vi "Save-Load Non-profile values.vi"(6 "Which file? (User profile.ini)":T1=enum."Loaded User profile.ini", 8 "error in":errorcluster, 11 "Function":T2=enum."Load from file") -> (0 "error out":errorcluster)   [LabVIEW 2017]
uses:
  Typedefs/Save-Load enum.ctl
  Typedefs/Which path.ctl
  <vilib>/Utility/config.llb/NI_LVConfig.lvlib
panel:
  out "any found?":bool
  out "all found?":bool
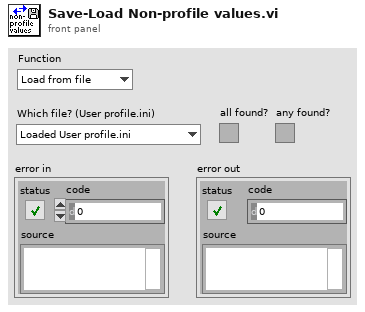
[diagram p1: front panel]
types:
  T1 = typedef "Which path.ctl" = enum16{"Configuration Files", "Calibration Files", "Images", "Setup.ini", "Loaded User profile.ini", "User's-Previous session.ini", "New user profile.ini", "Selected User profile.ini", "User profiles folder", "Power meter scaling.txt", "FOV Cal.ini"}
  T2 = typedef "Save-Load enum.ctl" = enum16{"Save to file", "Load from file", "Compare from file"}
  T3 = typedef "NI_LVConfig.lvlib/Config Data RefNum.ctl" = refnum<k1>
  T4 = typedef "Non-profile parameters cluster.ctl" = cluster{"Laser wavelength (nm)-When profile was saved":dbl}
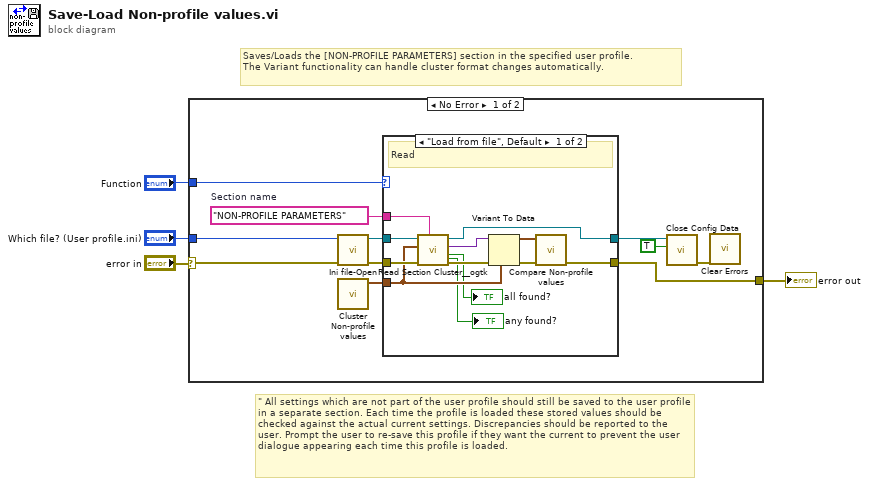
[diagram p0: block diagram]
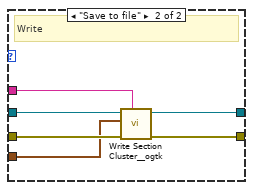
[diagram p2: hidden frame]
diagram:
  # "\"\tAll settings which are not part of the user profile should still be saved to the user profile in a separate section. Each time the profile is loaded these stored values should be checked against the actual current settings. Discrepancies should be reported to the user. Prompt the user to re-save this profile if they want the current to prevent the user dialogue appearing each time this profile is loaded."
  # "Saves/Loads the [NON-PROFILE PARAMETERS] section in the specified user profile.\nThe Variant functionality can handle cluster format changes automatically."
  n1 = case shown="No Error" "error in" {
    selector: "error in" -> [w6 w34]
    tunnel: [w8 w34] -> w4
    tunnel: "Which file? (User profile.ini)" -> [w9 _]
    tunnel: "Function" -> [w5 _]
    frame No Error {
      w15 = "NON-PROFILE PARAMETERS"  # Section name
      n2 = call "Ini file-Open.vi"("Error In"=w6, "Which file?"=w9) -> ("error out"=w12:errorcluster, "User profile ini file ref"=w13:T3)  [unwired: 6 in, 2 out]
      n3 = call "Cluster Non-profile values.vi"() -> ("Non-profile parameters cluster"=w7:T4)  [unwired: 10 in, 1 out]
      n4 = case shown="\"Load from file\", Default" w5 {
        tunnel: [w18 w30] -> w8
        tunnel: [w17 w33] -> w11
        tunnel: w12 -> [w26 w31]
        tunnel: w13 -> [w27 w32]
        tunnel: w15 -> [w22 w29]
        tunnel: w7 -> [w23 w28]
        frame "Load from file", Default {
          # "Read"
          n5 = call <userlib>:"Read Section Cluster__ogtk.vi"("section (optional)"=w22, "error in (no error)"=w26, "Section Formatted Cluster Type"=w23, "refnum"=w27) -> ("error out"=w24:errorcluster, "all found?"=→"all found?":bool, "Section Formatted Cluster"=w25:variant, "dup refnum"=w17:T3, "any found?"=→"any found?":bool)  [unwired: 3 in]
          n6 = Variant To Data(error in=w24, type=w23, Variant=w25) -> (data=w16:T4, error out=w19:errorcluster)
          n7 = call "Compare Non-profile values.vi"("error in (no error)"=w19, "Non-profile parameter values"=w16) -> ("error out"=w18:errorcluster)  [unwired: 9 in]
        }
        frame "Save to file" {
          # "Write"
          n8 = call <userlib>:"Write Section Cluster__ogtk.vi"("section (optional)"=w29, "error in (no error)"=w31, "Section Formatted Cluster"=w28, "refnum"=w32) -> ("error out"=w30:errorcluster, "dup refnum"=w33:T3)  [unwired: 6 in]
        }
      }
      n9 = call <vilib>:"Close Config Data.vi"("write file if changed (T)"=TRUE ("write configuration file? (F)"), "refnum"=w11) -> ("error out"=w10:errorcluster)  [unwired: 8 in, 1 out]
      n10 = call <vilib>:"Clear Errors.vi"("error in (no error)"=w10) -> ()  [unwired: 5 in, 2 out]
    }
    frame Error {
    }
  }
  "error out" <- w4
